vi "Create Power Supply.vi"(8 "error in":errorcluster) -> (0 "error out":errorcluster, 3 "Power Supply Interface out":refnum<class "PowerSupply.lvclass">)   [LabVIEW 2025, in "Power Supply.lvlib"]
uses:
  Power Supply.lvlib
  labview-plugins/PowerSupplies/PowerSupply/PowerSupply.lvlibp/PowerSupply/PowerSupply.lvclass
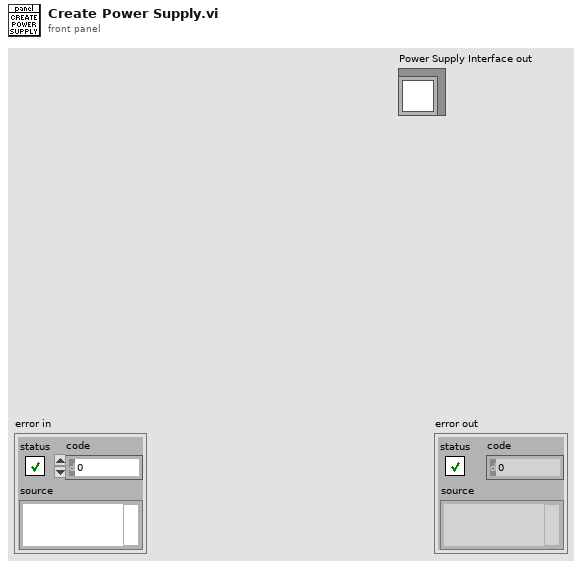
[diagram p1: front panel]
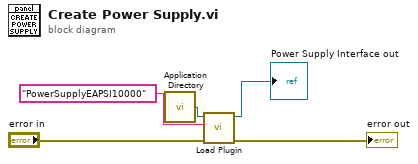
[diagram p0: block diagram]
diagram:
  n1 = call <vilib>:"Application Directory.vi"() -> ("Application Directory"=w5:path)
  n2 = call "Load Plugin.vi"("error in"="error in", "Plugin Name"="PowerSupplyEAPSI10000", "Application Directory"=w5) -> ("error out"=→"error out":errorcluster, "Power Supply Interface out"=→"Power Supply Interface out":refnum<class "PowerSupply.lvclass">)  [unwired: 7 in]
